vi "1.2.vi"() -> ()   [LabVIEW 2017]
panel:
  out "Numeric 2":dbl
  in  "Numeric":dbl
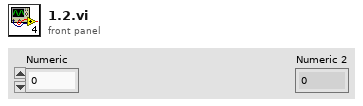
[diagram p1: front panel]
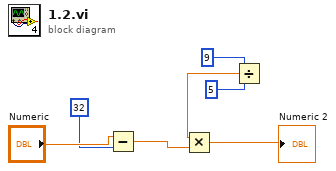
[diagram p0: block diagram]
diagram:
  n1 = Subtract(x="Numeric", y=32) -> (x-y=w7:dbl)
  n2 = Divide(x=5, y=9) -> (x/y=w6:dbl)
  n3 = Multiply(x=w6, y=w7) -> (x*y=→"Numeric 2":dbl)
